vi "test_without_gen.vi"() -> ()   [LabVIEW 2022 SP3]
uses:
  <vilib>/Analysis/Matrix/Datatypes/RealMatrix.ctl
  <vilib>/Utility/file.llb/Write Delimited Spreadsheet (DBL).vi
  <vilib>/Analysis/Matrix/NI_Matrix.lvlib
panel:
  out "output array":dbl[][](array[numeric])
  out "Array":dbl[](array[numeric])
  out "Real Matrix 2":T1
  out "Response 3":string
  out "Response 2":string
  out "Response":string
  in  "init":bool
  in  "meas":bool
  out "Numeric":dbl
  in  "Calibration points":T2(array[ring])
  in  "Number of measurements for each calibration point [max 20]":i32=5
  out "appended array":dbl[](array[numeric])
  in  "oscilloscope  Siglent SDS1102X+":refnum<visa-resource-name>="COM1"
  in  "stop":bool
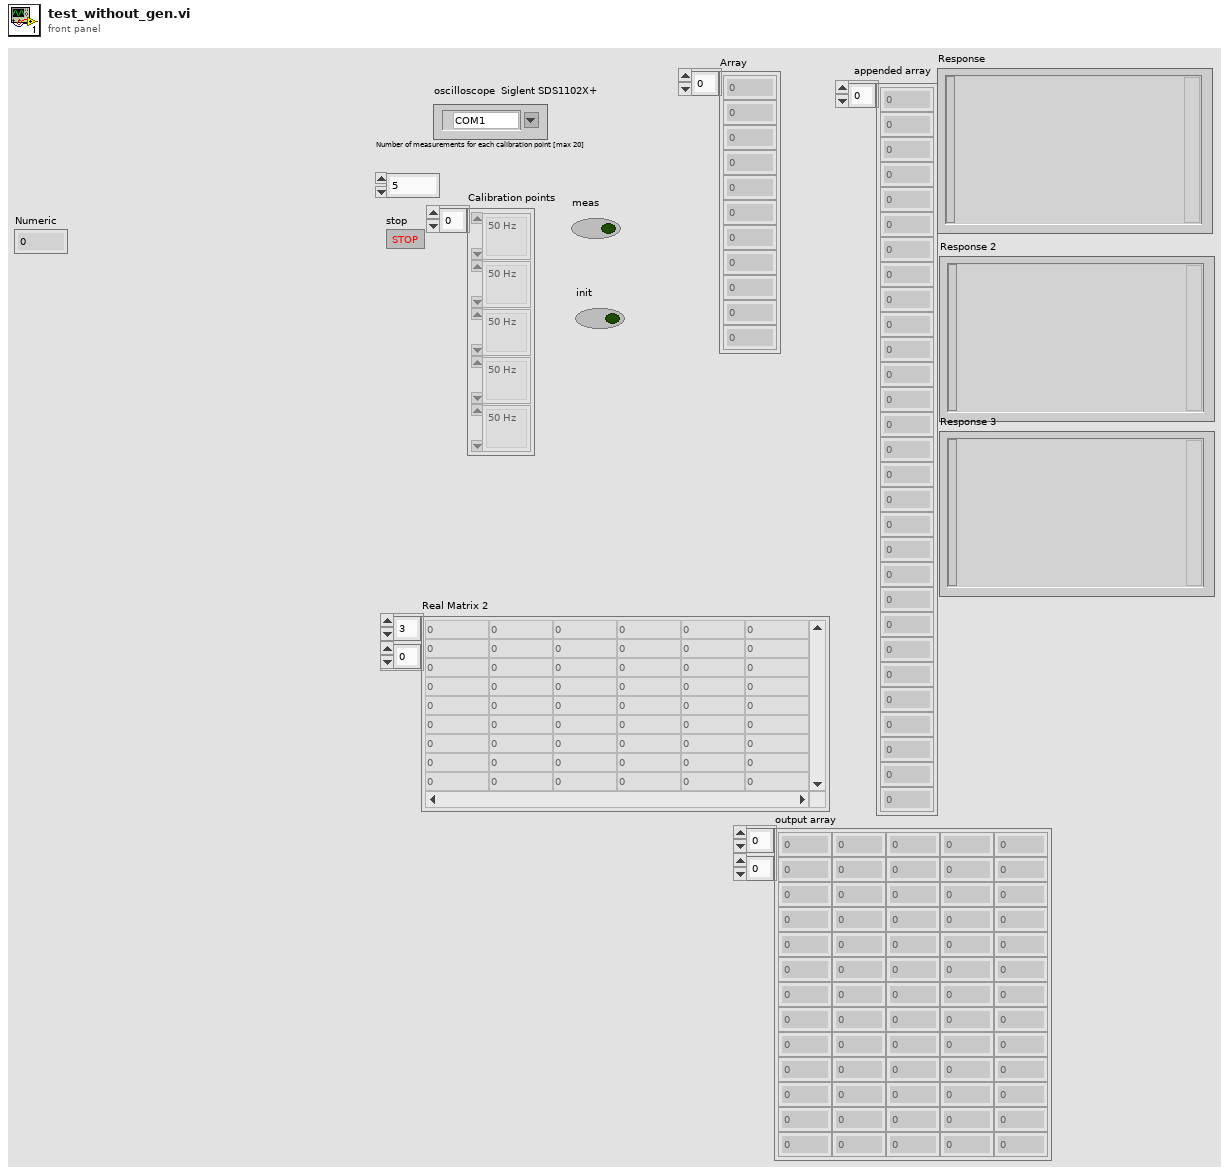
[diagram p1: front panel]
types:
  T1 = typedef "NI_Matrix.lvlib/RealMatrix.ctl" = dbl[][]
  T2 = enum16{"50 Hz", "1 kHz", "5 kHz", "20 kHz", "50 kHz", "100 kHz"}[]
  T3 = enum16{"50 Hz", "1 kHz", "5 kHz", "20 kHz", "50 kHz", "100 kHz"}
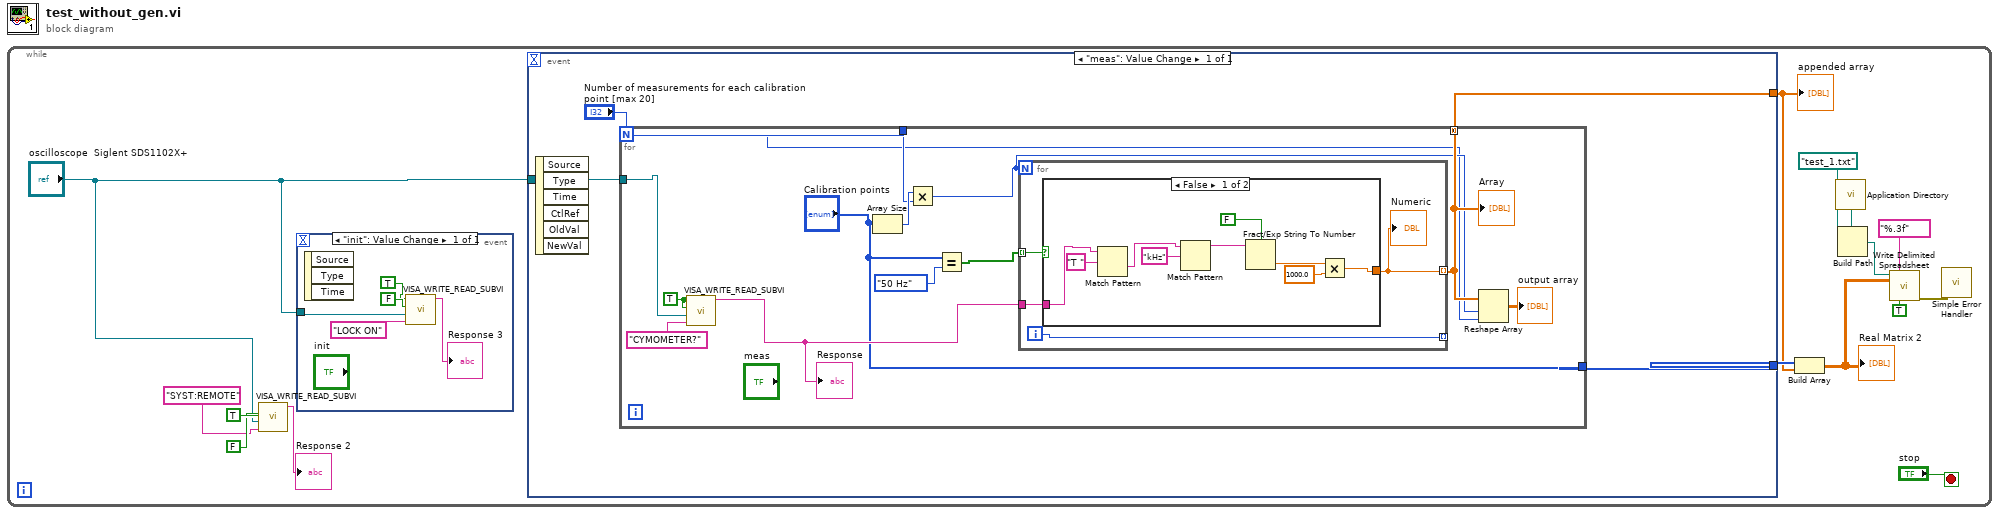
[diagram p0: block diagram]
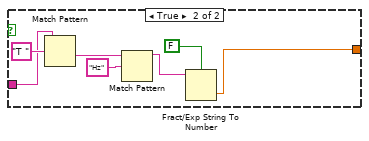
[diagram p2: hidden frame]
diagram:
  n1 = while {
    stop <- "stop" stop-if-true
    n2 = call "VISA_WRITE_READ_SUBVI.vi"("Command"="SYST:REMOTE", "VISA resource name"="oscilloscope  Siglent SDS1102X+", "Read 2"=FALSE ("Read"), "Write 2"=TRUE ("Write")) -> ("Response"=→"Response 2":string)  [unwired: 3 in, 1 out]
    n3 = event shown="[0] \"init\": Value Change" {
      selector: _ -> [_]
      dyn-events: _ -> [_]
      timeout: _ -> [_]
      tunnel: "oscilloscope  Siglent SDS1102X+" -> [w19]
      event "init": Value Change {
        n4 = event-data() -> ()  [unwired: 1 in, 3 out]
        n5 = call "VISA_WRITE_READ_SUBVI.vi"("Command"="LOCK ON", "VISA resource name"=w19, "Read 2"=FALSE ("Read"), "Write 2"=TRUE ("Write")) -> ("Response"=→"Response 3":string)  [unwired: 3 in, 1 out]
      }
    }
    n6 = event shown="[0] \"meas\": Value Change" {
      selector: _ -> [_]
      dyn-events: _ -> [_]
      timeout: _ -> [_]
      tunnel: "oscilloscope  Siglent SDS1102X+" -> [w24]
      tunnel: [w23] -> w2
      tunnel: [w21] -> w1
      event "meas": Value Change {
        n7 = event-data() -> ()  [unwired: 1 in, 6 out]
        n8 = for {
          N: "Number of measurements for each calibration point [max 20]" -> [w26]
          tunnel: w24 -> [w31]
          tunnel: [w28] -> w21 mode=concatenating
          tunnel: "Number of measurements for each calibration point [max 20]" -> [w30]
          tunnel: ["Calibration points"] -> w23
          w33 = TRUE ("Write 2")
          n9 = call "VISA_WRITE_READ_SUBVI.vi"("Command"="CYMOMETER?", "VISA resource name"=w31, "Read 2"=w33, "Write 2"=w33) -> ("Response"=w37:string)  [unwired: 3 in, 1 out]
          "Response" <- w37
          n10 = Array Size(array="Calibration points") -> (size(s)=w35:i32)
          n11 = Multiply(x=w35, y=w30) -> (x*y=w27:i32)
          n12 = Equal?(x="Calibration points", y=T3."50 Hz" ("Bod 1")) -> (x = y?=w36:bool[])
          n13 = for {
            N: w27 -> [_]
            tunnel: w36 -> [w41] mode=indexing
            tunnel: [w40] -> w28 mode=indexing
            tunnel: w37 -> [w39]
            tunnel: [w38] -> _ mode=indexing
            i -> [w38]
            n14 = case shown="False" w41 {
              tunnel: [w44 w52] -> w40
              tunnel: w39 -> [w42 w51]
              frame False {
                n15 = Match Pattern(string=w42, regular expression="T ") -> (after substring=w49:string)  [unwired: 1 in, 3 out]
                n16 = Match Pattern(string=w49, regular expression="kHz") -> (before substring=w47:string)  [unwired: 1 in, 3 out]
                n17 = Fract/Exp String To Number(use system decimal point (T)=FALSE, string=w47) -> (number=w45:dbl)  [unwired: 2 in, 1 out]
                n18 = Multiply(x=w45, y=1000.0) -> (x*y=w44:dbl)
              }
              frame True {
                n19 = Match Pattern(string=w51, regular expression="T ") -> (after substring=w56:string)  [unwired: 1 in, 3 out]
                n20 = Match Pattern(string=w56, regular expression="Hz") -> (before substring=w54:string)  [unwired: 1 in, 3 out]
                n21 = Fract/Exp String To Number(use system decimal point (T)=FALSE, string=w54) -> (number=w52:dbl)  [unwired: 2 in, 1 out]
              }
            }
            "Numeric" <- w40
          }
          "Array" <- w28
          n22 = Reshape Array(w28, w27, w26) -> (→"output array":dbl[][])
        }
      }
    }
    "appended array" <- w1
    n23 = Build Array(w2, w1) -> (w4:dbl[][])
    "Real Matrix 2" <- w4
    n24 = call <vilib>:"Application Directory.vi"() -> ("Application Directory"=w7:path)
    n25 = Build Path(base path=w7, name or relative path=path "test_1.txt") -> (appended path=w6:path)
    n26 = call-poly <vilib>:"Write Delimited Spreadsheet.vi"("file path (dialog if empty)"=w6, "format (%.3f)"="%.3f", "2D data"=w4, "transpose? (no:F)"=TRUE) -> ("error out"=w9:errorcluster)  [unwired: 10 in, 1 out]
    n27 = call <vilib>:"Simple Error Handler.vi"("error in (no error)"=w9) -> ()  [unwired: 4 in, 5 out]
  }
